vi "StartFindHome.vi"(8 "error in (no error)":errorcluster, 9 "Axis (1..4)":T1=1 items=["X"=1, "Y"=2, "Z"=3, "T"=4], 10 "Absolute 0 position, mm":dbl=5000.0 caption="Absolute 0 position from limit switch, mm", 11 "VXMx2 in":refnum<class "VXMx2.lvclass">) -> (0 "error out":errorcluster, 3 "VXMx2 out":refnum<class "VXMx2.lvclass">)   [LabVIEW 2018, in "VXMx2.lvclass"]
doc: "For one axis, send commands that find limit switch and establish home position and zero.\nBut don't wait for motion to complete."
uses:
  VXMx2.lvclass
  <instrlib>/Velmex VXM/Public/VXM Axis.ctl
  VXMx2.lvclass/VXMx2.ctl
  <instrlib>/Velmex VXM/Velmex VXM.lvlib
panel:
  # "THIS IS NOT A GENERAL USE VI, \nit sets home relative to a limit switch"
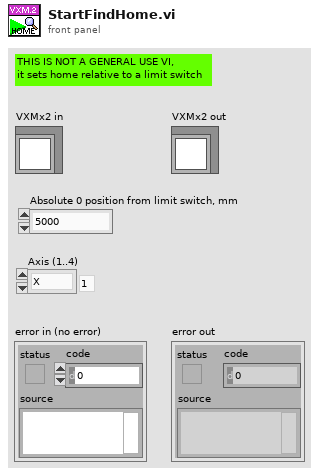
[diagram p1: front panel]
types:
  T1 = typedef "Velmex VXM.lvlib/VXM Axis.ctl" = u16
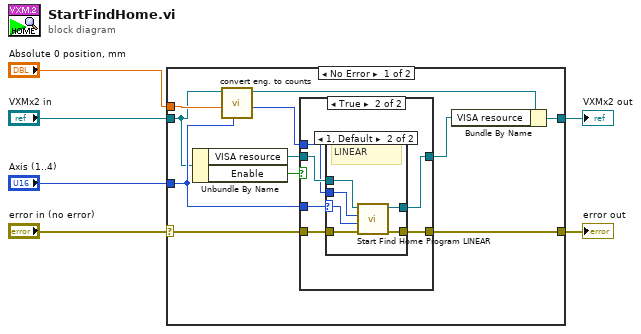
[diagram p0: block diagram]
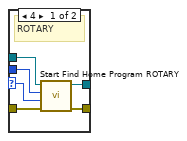
[diagram p3: hidden frame]
diagram:
  n1 = case shown="No Error" "error in (no error)" {
    selector: "error in (no error)" -> [w16 w39]
    tunnel: [w15 w39] -> w5
    tunnel: [w14 w38] -> w3
    tunnel: "VXMx2 in" -> [w8 w38]
    tunnel: "Absolute 0 position, mm" -> [w10 _]
    tunnel: "Axis (1..4)" -> [w11 _]
    frame No Error {
      n2 = Unbundle By Name(w8) -> ("VISA resource"=w17:refnum<visa-resource-name>, "Enable"=w12:bool)
      n3 = call "convert eng. to counts.vi"("Axis (1..4)"=w11, "Position, eng units"=w10, "VXMx2 in"=w8) -> ("Position, counts"=w9:i32, "VXMx2 out"=w7:refnum<class "VXMx2.lvclass">)  [unwired: 5 in, 2 out]
      n4 = case shown="True" w12 {
        tunnel: w9 -> [_ w21]
        tunnel: w11 -> [_ w20]
        tunnel: w17 -> [w19 w25]
        tunnel: w16 -> [w18 w24]
        tunnel: [w18 w23] -> w15
        tunnel: [w19 w22] -> w13
        frame False {
        }
        frame True {
          n5 = case shown="1, Default" w20 {
            selector: w20 -> [w26 w32]
            tunnel: w25 -> [w29 w34]
            tunnel: w24 -> [w30 w37]
            tunnel: [w31 w36] -> w23
            tunnel: [w28 w35] -> w22
            tunnel: w21 -> [w27 w33]
            frame 4 {
              # "ROTARY"
              n6 = call <instrlib>:"Start Find Home Program ROTARY.vi"("error in (no error)"=w30, "Axis (1..4)"=w26, "Homing compensation"=w27, "VISA resource name"=w29) -> ("error out"=w31:errorcluster, "VISA resource out"=w28:refnum<visa-resource-name>)  [unwired: 6 in]
            }
            frame 1, Default {
              # "LINEAR"
              n7 = call <instrlib>:"Start Find Home Program LINEAR.vi"("error in (no error)"=w37, "Axis (1..4)"=w32, "Absolute 0 position, counts"=w33, "VISA resource name"=w34) -> ("error out"=w36:errorcluster, "VISA resource out"=w35:refnum<visa-resource-name>)  [unwired: 6 in]
            }
          }
        }
      }
      n8 = Bundle By Name(cluster=w7, "VISA resource"=w13) -> (w14:refnum<class "VXMx2.lvclass">)
    }
    frame Error {
    }
  }
  "error out" <- w5
  "VXMx2 out" <- w3
